vi "每个元素都写入临时表格 (子VI).vi"(8 "error in (no error)":errorcluster caption="错误输入（无错误）", 11 "组合框":string(combo)) -> (0 "error out":errorcluster caption="错误输出")   [LabVIEW 2016, in "数据传输系统.lvlib"]
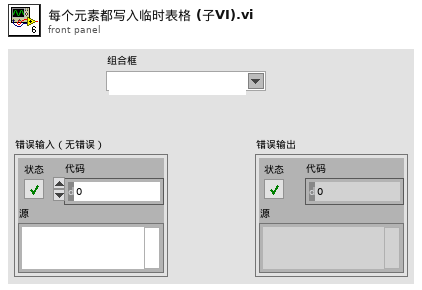
[diagram p1: front panel]
types:
  T1 = enum16{"CODMn", "PH", "氨氮", "总氮", "总磷", "CODCr", "电导率", "水温", "DO", "浊度", "叶绿素", "藻密度"}
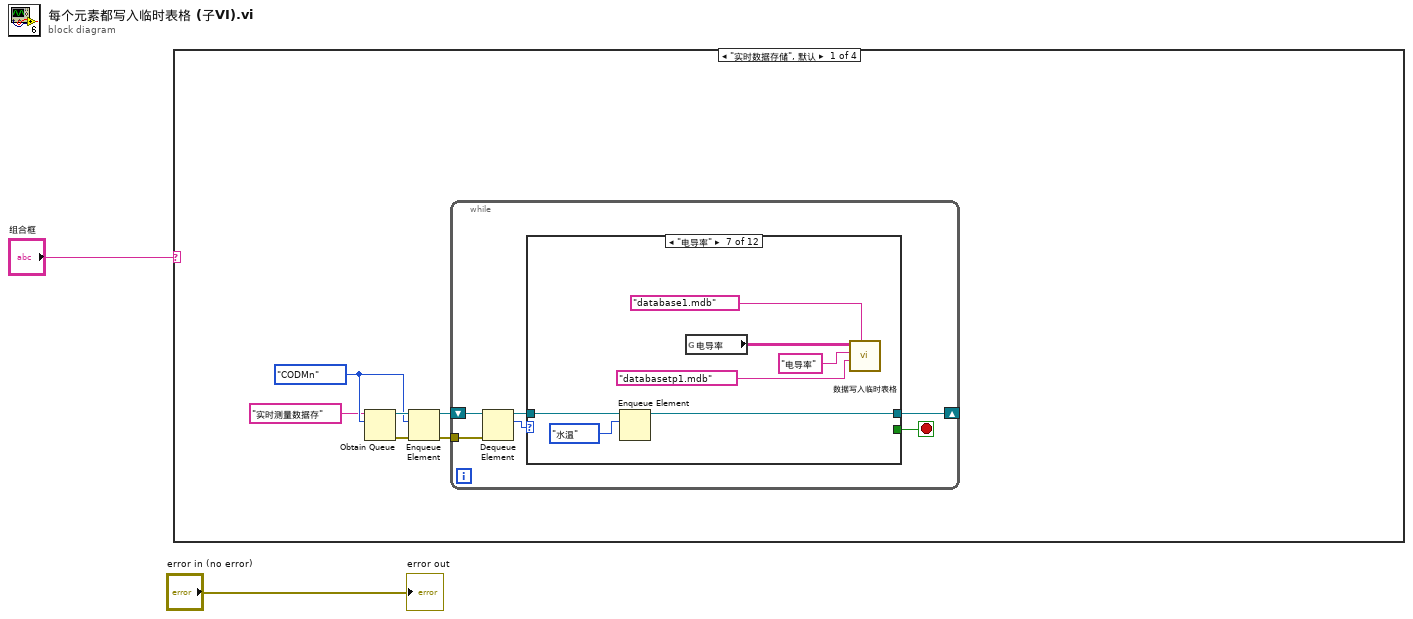
[diagram p0: block diagram]
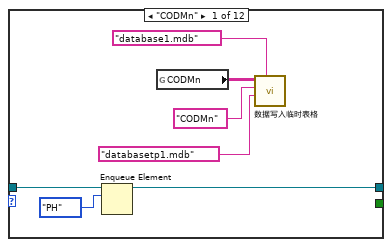
[diagram p2: hidden frame]
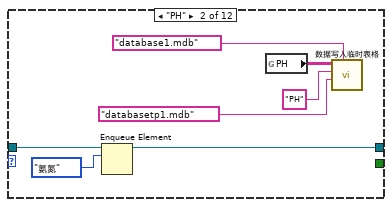
[diagram p3: hidden frame]
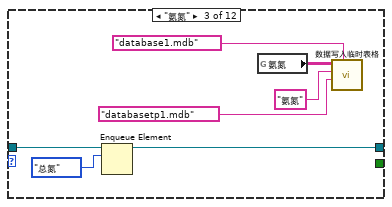
[diagram p4: hidden frame]
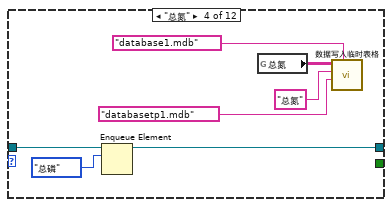
[diagram p5: hidden frame]
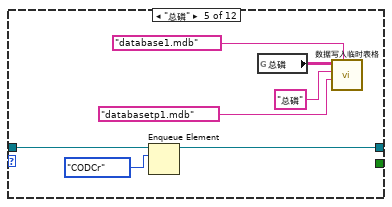
[diagram p6: hidden frame]
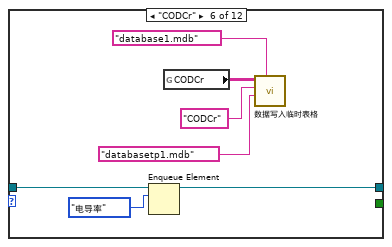
[diagram p7: hidden frame]
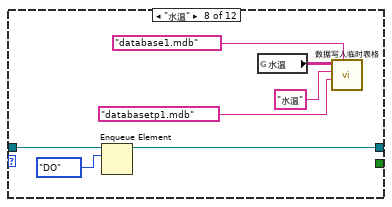
[diagram p8: hidden frame]
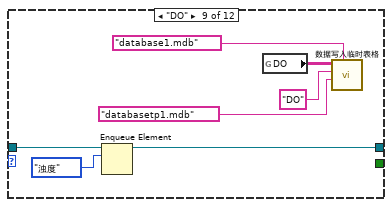
[diagram p9: hidden frame]
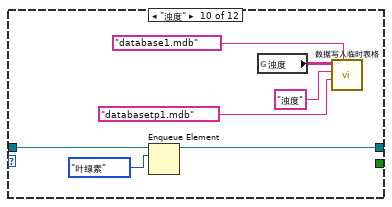
[diagram p10: hidden frame]
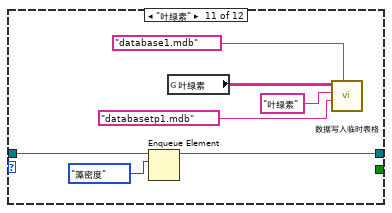
[diagram p11: hidden frame]
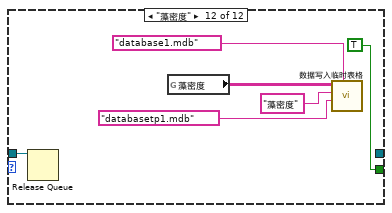
[diagram p12: hidden frame]
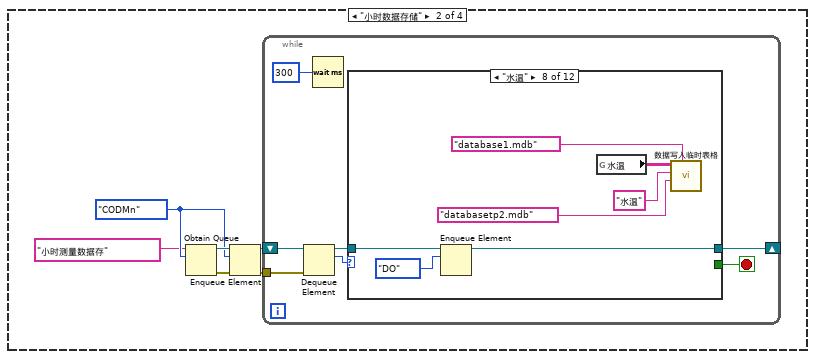
[diagram p13: hidden frame]
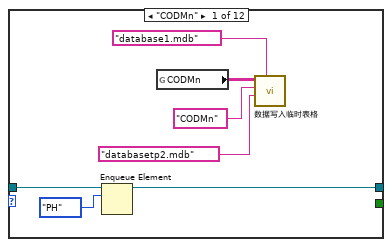
[diagram p14: hidden frame]
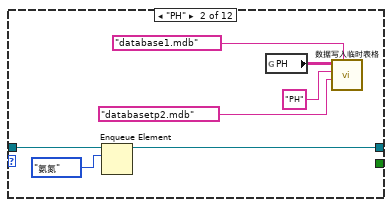
[diagram p15: hidden frame]
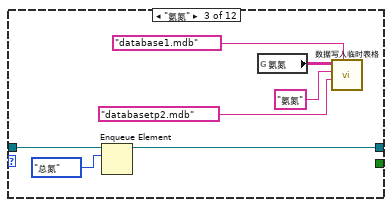
[diagram p16: hidden frame]
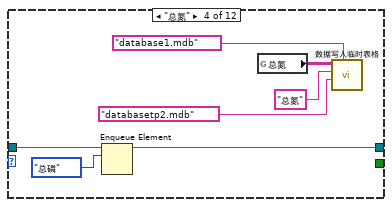
[diagram p17: hidden frame]
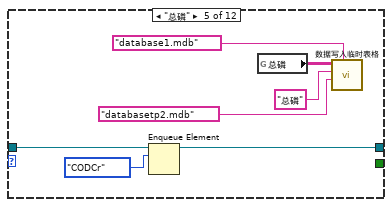
[diagram p18: hidden frame]
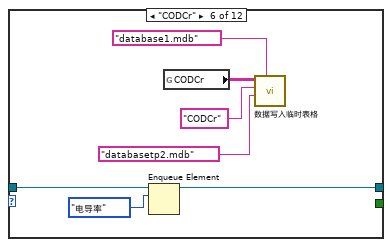
[diagram p19: hidden frame]
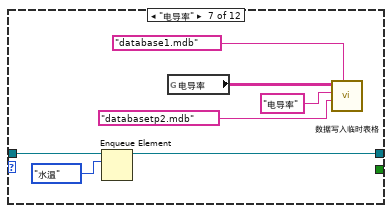
[diagram p20: hidden frame]
diagram:
  n1 = case shown="\"实时数据存储\", 默认" "组合框" {
    frame "实时数据存储", Default {
      w4 = T1."CODMn"
      n2 = Obtain Queue(name (unnamed)="实时测量数据存" ("新元素/子数组"), element data type=w4) -> (queue out=w8:refnum<queue>, error out=w5:errorcluster)  [unwired: 3 in, 1 out]
      n3 = Enqueue Element(queue=w8, element=w4, error in (no error)=w5) -> (queue out=w7:refnum<queue>, error out=w6:errorcluster)  [unwired: 1 in, 1 out]
      n4 = while {
        shift-right: [w12] -> _
        shift-left: w7 -> [w14]
        tunnel: w6 -> [w11]
        stop <- w9 stop-if-true
        n5 = Dequeue Element(queue=w14, error in (no error)=w11) -> (queue out=w13:refnum<queue>, element=w10:T1)  [unwired: 1 in, 2 out]
        n6 = case shown="\"电导率\"" w10 {
          tunnel: w13 -> [w21 w28 w34 w42 w48 w55 w62 w69 w76 w83 w90 w96]
          tunnel: [w20 w27 w35 w41 w47 w54 w61 w68 w75 w82 w89 _] -> w12
          tunnel: [_ _ _ _ _ _ _ _ _ _ _ TRUE] -> w9
          frame "CODMn" {
            n7 = Enqueue Element(queue=w21, element=T1."PH") -> (queue out=w20:refnum<queue>)  [unwired: 2 in, 2 out]
            n8 = global read "全局 所有参数.vi" "CODMn"() -> (w17:string[][])
            n9 = call "数据写入临时表格.vi"("表格选择"="database1.mdb", "存储表格"="databasetp1.mdb", "table"="CODMn" ("元素"), "data"=w17) -> ()  [unwired: 7 in, 1 out]
          }
          frame "PH" {
            n10 = Enqueue Element(queue=w28, element=T1."氨氮") -> (queue out=w27:refnum<queue>)  [unwired: 2 in, 2 out]
            n11 = global read "全局 所有参数.vi" "PH"() -> (w25:string[][])
            n12 = call "数据写入临时表格.vi"("表格选择"="database1.mdb", "存储表格"="databasetp1.mdb", "table"="PH" ("元素"), "data"=w25) -> ()  [unwired: 7 in, 1 out]
          }
          frame "氨氮" {
            n13 = Enqueue Element(queue=w34, element=T1."总氮") -> (queue out=w35:refnum<queue>)  [unwired: 2 in, 2 out]
            n14 = global read "全局 所有参数.vi" "氨氮"() -> (w32:string[][])
            n15 = call "数据写入临时表格.vi"("表格选择"="database1.mdb", "存储表格"="databasetp1.mdb", "table"="氨氮", "data"=w32) -> ()  [unwired: 7 in, 1 out]
          }
          frame "总氮" {
            n16 = Enqueue Element(queue=w42, element=T1."总磷") -> (queue out=w41:refnum<queue>)  [unwired: 2 in, 2 out]
            n17 = global read "全局 所有参数.vi" "总氮"() -> (w39:string[][])
            n18 = call "数据写入临时表格.vi"("表格选择"="database1.mdb", "存储表格"="databasetp1.mdb", "table"="总氮" ("元素"), "data"=w39) -> ()  [unwired: 7 in, 1 out]
          }
          frame "总磷" {
            n19 = Enqueue Element(queue=w48, element=T1."CODCr") -> (queue out=w47:refnum<queue>)  [unwired: 2 in, 2 out]
            n20 = global read "全局 所有参数.vi" "总磷"() -> (w46:string[][])
            n21 = call "数据写入临时表格.vi"("表格选择"="database1.mdb", "存储表格"="databasetp1.mdb", "table"="总磷" ("元素"), "data"=w46) -> ()  [unwired: 7 in, 1 out]
          }
          frame "CODCr" {
            n22 = Enqueue Element(queue=w55, element=T1."电导率") -> (queue out=w54:refnum<queue>)  [unwired: 2 in, 2 out]
            n23 = global read "全局 所有参数.vi" "CODCr"() -> (w53:string[][])
            n24 = call "数据写入临时表格.vi"("表格选择"="database1.mdb", "存储表格"="databasetp1.mdb", "table"="CODCr" ("元素"), "data"=w53) -> ()  [unwired: 7 in, 1 out]
          }
          frame "电导率" {
            n25 = Enqueue Element(queue=w62, element=T1."水温") -> (queue out=w61:refnum<queue>)  [unwired: 2 in, 2 out]
            n26 = global read "全局 所有参数.vi" "电导率"() -> (w60:string[][])
            n27 = call "数据写入临时表格.vi"("表格选择"="database1.mdb", "存储表格"="databasetp1.mdb", "table"="电导率" ("元素"), "data"=w60) -> ()  [unwired: 7 in, 1 out]
          }
          frame "水温" {
            n28 = Enqueue Element(queue=w69, element=T1."DO") -> (queue out=w68:refnum<queue>)  [unwired: 2 in, 2 out]
            n29 = global read "全局 所有参数.vi" "水温"() -> (w67:string[][])
            n30 = call "数据写入临时表格.vi"("表格选择"="database1.mdb", "存储表格"="databasetp1.mdb", "table"="水温" ("元素"), "data"=w67) -> ()  [unwired: 7 in, 1 out]
          }
          frame "DO" {
            n31 = Enqueue Element(queue=w76, element=T1."浊度") -> (queue out=w75:refnum<queue>)  [unwired: 2 in, 2 out]
            n32 = global read "全局 所有参数.vi" "DO"() -> (w74:string[][])
            n33 = call "数据写入临时表格.vi"("表格选择"="database1.mdb", "存储表格"="databasetp1.mdb", "table"="DO" ("元素"), "data"=w74) -> ()  [unwired: 7 in, 1 out]
          }
          frame "浊度" {
            n34 = Enqueue Element(queue=w83, element=T1."叶绿素") -> (queue out=w82:refnum<queue>)  [unwired: 2 in, 2 out]
            n35 = global read "全局 所有参数.vi" "浊度"() -> (w81:string[][])
            n36 = call "数据写入临时表格.vi"("表格选择"="database1.mdb", "存储表格"="databasetp1.mdb", "table"="浊度" ("元素"), "data"=w81) -> ()  [unwired: 7 in, 1 out]
          }
          frame "叶绿素" {
            n37 = Enqueue Element(queue=w90, element=T1."藻密度") -> (queue out=w89:refnum<queue>)  [unwired: 2 in, 2 out]
            n38 = global read "全局 所有参数.vi" "叶绿素"() -> (w88:string[][])
            n39 = call "数据写入临时表格.vi"("表格选择"="database1.mdb", "存储表格"="databasetp1.mdb", "table"="叶绿素" ("元素"), "data"=w88) -> ()  [unwired: 7 in, 1 out]
          }
          frame "藻密度" {
            n40 = Release Queue(queue=w96) -> ()  [unwired: 2 in, 3 out]
            n41 = global read "全局 所有参数.vi" "藻密度"() -> (w95:string[][])
            n42 = call "数据写入临时表格.vi"("表格选择"="database1.mdb", "存储表格"="databasetp1.mdb", "table"="藻密度" ("元素"), "data"=w95) -> ()  [unwired: 7 in, 1 out]
          }
        }
      }
    }
    frame "小时数据存储" {
      w99 = T1."CODMn"
      n43 = Obtain Queue(name (unnamed)="小时测量数据存" ("新元素/子数组"), element data type=w99) -> (queue out=w103:refnum<queue>, error out=w100:errorcluster)  [unwired: 3 in, 1 out]
      n44 = Enqueue Element(queue=w103, element=w99, error in (no error)=w100) -> (queue out=w102:refnum<queue>, error out=w101:errorcluster)  [unwired: 1 in, 1 out]
      n45 = while {
        shift-right: [w108] -> _
        shift-left: w102 -> [w110]
        tunnel: w101 -> [w107]
        stop <- w105 stop-if-true
        n46 = Dequeue Element(queue=w110, error in (no error)=w107) -> (queue out=w109:refnum<queue>, element=w106:T1)  [unwired: 1 in, 2 out]
        n47 = Wait (ms)(milliseconds to wait=u32 300 ("等待时间（毫秒）")) -> ()  [unwired: 1 out]
        n48 = case shown="\"水温\"" w106 {
          tunnel: w109 -> [w117 w124 w130 w138 w144 w151 w158 w165 w172 w179 w186 w192]
          tunnel: [w116 w123 w131 w137 w143 w150 w157 w164 w171 w178 w185 _] -> w108
          tunnel: [_ _ _ _ _ _ _ _ _ _ _ TRUE] -> w105
          frame "CODMn" {
            n49 = Enqueue Element(queue=w117, element=T1."PH") -> (queue out=w116:refnum<queue>)  [unwired: 2 in, 2 out]
            n50 = global read "全局 所有参数.vi" "CODMn"() -> (w113:string[][])
            n51 = call "数据写入临时表格.vi"("表格选择"="database1.mdb", "存储表格"="databasetp2.mdb", "table"="CODMn" ("元素"), "data"=w113) -> ()  [unwired: 7 in, 1 out]
          }
          frame "PH" {
            n52 = Enqueue Element(queue=w124, element=T1."氨氮") -> (queue out=w123:refnum<queue>)  [unwired: 2 in, 2 out]
            n53 = global read "全局 所有参数.vi" "PH"() -> (w121:string[][])
            n54 = call "数据写入临时表格.vi"("表格选择"="database1.mdb", "存储表格"="databasetp2.mdb", "table"="PH" ("元素"), "data"=w121) -> ()  [unwired: 7 in, 1 out]
          }
          frame "氨氮" {
            n55 = Enqueue Element(queue=w130, element=T1."总氮") -> (queue out=w131:refnum<queue>)  [unwired: 2 in, 2 out]
            n56 = global read "全局 所有参数.vi" "氨氮"() -> (w128:string[][])
            n57 = call "数据写入临时表格.vi"("表格选择"="database1.mdb", "存储表格"="databasetp2.mdb", "table"="氨氮", "data"=w128) -> ()  [unwired: 7 in, 1 out]
          }
          frame "总氮" {
            n58 = Enqueue Element(queue=w138, element=T1."总磷") -> (queue out=w137:refnum<queue>)  [unwired: 2 in, 2 out]
            n59 = global read "全局 所有参数.vi" "总氮"() -> (w135:string[][])
            n60 = call "数据写入临时表格.vi"("表格选择"="database1.mdb", "存储表格"="databasetp2.mdb", "table"="总氮" ("元素"), "data"=w135) -> ()  [unwired: 7 in, 1 out]
          }
          frame "总磷" {
            n61 = Enqueue Element(queue=w144, element=T1."CODCr") -> (queue out=w143:refnum<queue>)  [unwired: 2 in, 2 out]
            n62 = global read "全局 所有参数.vi" "总磷"() -> (w142:string[][])
            n63 = call "数据写入临时表格.vi"("表格选择"="database1.mdb", "存储表格"="databasetp2.mdb", "table"="总磷" ("元素"), "data"=w142) -> ()  [unwired: 7 in, 1 out]
          }
          frame "CODCr" {
            n64 = Enqueue Element(queue=w151, element=T1."电导率") -> (queue out=w150:refnum<queue>)  [unwired: 2 in, 2 out]
            n65 = global read "全局 所有参数.vi" "CODCr"() -> (w149:string[][])
            n66 = call "数据写入临时表格.vi"("表格选择"="database1.mdb", "存储表格"="databasetp2.mdb", "table"="CODCr" ("元素"), "data"=w149) -> ()  [unwired: 7 in, 1 out]
          }
          frame "电导率" {
            n67 = Enqueue Element(queue=w158, element=T1."水温") -> (queue out=w157:refnum<queue>)  [unwired: 2 in, 2 out]
            n68 = global read "全局 所有参数.vi" "电导率"() -> (w156:string[][])
            n69 = call "数据写入临时表格.vi"("表格选择"="database1.mdb", "存储表格"="databasetp2.mdb", "table"="电导率" ("元素"), "data"=w156) -> ()  [unwired: 7 in, 1 out]
          }
          frame "水温" {
            n70 = Enqueue Element(queue=w165, element=T1."DO") -> (queue out=w164:refnum<queue>)  [unwired: 2 in, 2 out]
            n71 = global read "全局 所有参数.vi" "水温"() -> (w163:string[][])
            n72 = call "数据写入临时表格.vi"("表格选择"="database1.mdb", "存储表格"="databasetp2.mdb", "table"="水温" ("元素"), "data"=w163) -> ()  [unwired: 7 in, 1 out]
          }
          frame "DO" {
            n73 = Enqueue Element(queue=w172, element=T1."浊度") -> (queue out=w171:refnum<queue>)  [unwired: 2 in, 2 out]
            n74 = global read "全局 所有参数.vi" "DO"() -> (w170:string[][])
            n75 = call "数据写入临时表格.vi"("表格选择"="database1.mdb", "存储表格"="databasetp2.mdb", "table"="DO" ("元素"), "data"=w170) -> ()  [unwired: 7 in, 1 out]
          }
          frame "浊度" {
            n76 = Enqueue Element(queue=w179, element=T1."叶绿素") -> (queue out=w178:refnum<queue>)  [unwired: 2 in, 2 out]
            n77 = global read "全局 所有参数.vi" "浊度"() -> (w177:string[][])
            n78 = call "数据写入临时表格.vi"("表格选择"="database1.mdb", "存储表格"="databasetp2.mdb", "table"="浊度" ("元素"), "data"=w177) -> ()  [unwired: 7 in, 1 out]
          }
          frame "叶绿素" {
            n79 = Enqueue Element(queue=w186, element=T1."藻密度") -> (queue out=w185:refnum<queue>)  [unwired: 2 in, 2 out]
            n80 = global read "全局 所有参数.vi" "叶绿素"() -> (w184:string[][])
            n81 = call "数据写入临时表格.vi"("表格选择"="database1.mdb", "存储表格"="databasetp2.mdb", "table"="叶绿素" ("元素"), "data"=w184) -> ()  [unwired: 7 in, 1 out]
          }
          frame "藻密度" {
            n82 = Release Queue(queue=w192) -> ()  [unwired: 2 in, 3 out]
            n83 = global read "全局 所有参数.vi" "藻密度"() -> (w191:string[][])
            n84 = call "数据写入临时表格.vi"("表格选择"="database1.mdb", "存储表格"="databasetp2.mdb", "table"="藻密度" ("元素"), "data"=w191) -> ()  [unwired: 7 in, 1 out]
          }
        }
      }
    }
    frame "日志信息存储" {
      n85 = call "数据表比对.vi"("table输入"="操作日志存表 ") -> ("error out"=w195:errorcluster, "待发送数据"=w199:string[][])  [unwired: 7 in, 2 out]
      n86 = call "数据写入临时表格.vi"("表格选择"="database3.mdb", "error in"=w195, "存储表格"="databasetp3.mdb", "table"="操作日志", "data"=w199) -> ()  [unwired: 6 in, 1 out]
    }
    frame "报警信息存储" {
      n87 = call "数据表比对.vi"("table输入"="报警信息存表 ") -> ("error out"=w201:errorcluster, "待发送数据"=w205:string[][])  [unwired: 7 in, 2 out]
      n88 = call "数据写入临时表格.vi"("表格选择"="database3.mdb", "error in"=w201, "存储表格"="databasetp3.mdb", "table"="报警信息", "data"=w205) -> ()  [unwired: 6 in, 1 out]
    }
  }
  "error out" <- "error in (no error)"
